vi "Create metadata Tag Cluster.vi"(2 "Count":u32, 3 "Tag to store\nmetadata in\n(ImageID tag)":u16, 4 "Byte stream offset\nwhere tag should have been":i32, 5 "Byte stream offset\nwhere data should be":u32) -> (0 "Cluster":T1, 1 "Insert tag before inserting data?":bool)   [LabVIEW 2015, in "Tiff reader.lvlib"]
doc: "Create the metadata cluster."
uses:
  Tiff reader.lvlib
  FieldTypes.ctl
  IFD Entry.ctl
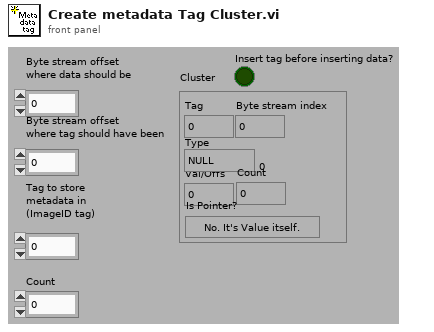
[diagram p1: front panel]
types:
  T1 = typedef "Tiff reader.lvlib/IFD Entry.ctl" = cluster{"Tag":u16, "Type":T2, "Count":u32, "Val/Offs":u32, "Is Pointer?":bool, "Byte stream index":i32}
  T2 = typedef "Tiff reader.lvlib/FieldTypes.ctl" = enum16{"NULL", "U8", "ASCII7", "U16", "U32", "RATIONAL", "SByte(I8)", "Undef(8Bit)", "I16", "I32", "SRat(4B:4B)", "SGL(4Byte)", "DBL(8Byte)"}
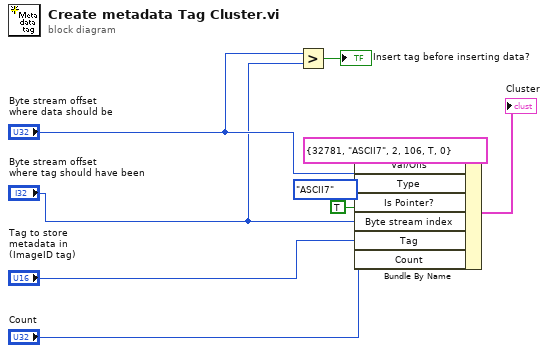
[diagram p0: block diagram]
diagram:
  n1 = Greater?(x="Byte stream offset\nwhere data should be", y="Byte stream offset\nwhere tag should have been") -> (0:→"Insert tag before inserting data?":bool)
  n2 = Bundle By Name(cluster=T1 {"Tag"=32781, "Type"=enum."ASCII7", "Count"=2, "Val/Offs"=106, "Is Pointer?"=TRUE, "Byte stream index"=0} ("Cluster"), "Val/Offs"="Byte stream offset\nwhere data should be", "Type"=FieldTypes."ASCII7", "Is Pointer?"=TRUE ("Is Val/Offs(T)"), "Byte stream index"="Byte stream offset\nwhere tag should have been", "Tag"="Tag to store\nmetadata in\n(ImageID tag)", "Count"="Count") -> (→"Cluster":T1)
